vi "Cleanup.vi"(8 "error in (no error)":errorcluster, 11 "Tester in":refnum<class "Tester.lvclass">) -> (0 "error out":errorcluster)   [LabVIEW 2020, in "Tester.lvlib" / "Tester.lvclass"]
uses:
  Tester.lvclass
  Tester.lvclass/Tester.ctl
  Results/Results.lvclass
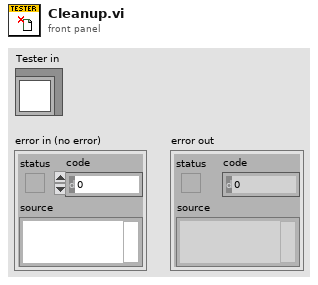
[diagram p1: front panel]
types:
  T1 = typedef "Tester.lvlib/Tester.lvclass/Execution Ref.ctl" = cluster{"Sequence":refnum<class "Sequence.lvclass">, "Step":i32, "Results":refnum<class "Results.lvclass">, "State":T2, "Run Step VI":refnum<vi>, "Abort":bool}
  T2 = typedef "Tester.lvlib/Tester.lvclass/State.ctl" = enum16{"Idle", "In Progress", "Completed"}
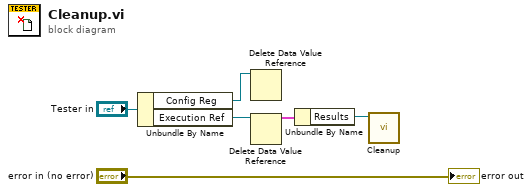
[diagram p0: block diagram]
diagram:
  n1 = Unbundle By Name("Tester in") -> ("Config Reg"=w3:refnum<data-value>, "Execution Ref"=w4:refnum<data-value>)
  n2 = Delete Data Value Reference(data value reference=w3) -> ()  [unwired: 1 in, 2 out]
  n3 = Delete Data Value Reference(data value reference=w4) -> (data value=w2:T1)  [unwired: 1 in, 1 out]
  n4 = Unbundle By Name(w2) -> ("Results"=w1:refnum<class "Results.lvclass">)
  n5 = call "Cleanup.vi"("Results in"=w1) -> ()  [unwired: 10 in, 1 out]
  "error out" <- "error in (no error)"
